vi "CIMAQ_ReadFile_UID.vi"   [LabVIEW 2017]
types:
  T1 = typedef "IMAQ Image.ctl" = refnum<image>
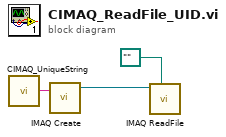
[diagram p0: block diagram]
diagram:
  n1 = call <userlib>:"CIMAQ_UniqueString.vi"() -> ("String"=w1:string)  [unwired: 5 in]
  n2 = call "IMAQ Create"("Image Name"=w1) -> ("New Image"=w2:T1)  [unwired: 4 in, 1 out]
  n3 = call "IMAQ ReadFile"("File Path"=path "", "Image"=w2) -> ()  [unwired: 5 in, 5 out]
